vi "Generate Rotation Matrix.vi"(1 "Angle":dbl) -> (0 "Rotation Matrix":T1)   [LabVIEW 2019, in "Referential.lvclass"]
uses:
  Referential.lvclass
  <vilib>/Analysis/Matrix/Datatypes/RealMatrix.ctl
  <vilib>/Analysis/Matrix/NI_Matrix.lvlib
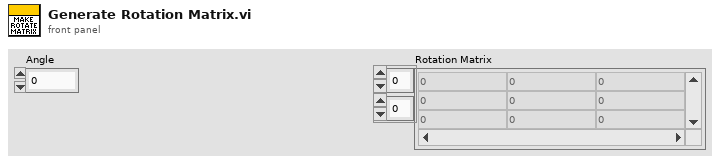
[diagram p1: front panel]
types:
  T1 = typedef "NI_Matrix.lvlib/RealMatrix.ctl" = dbl[][]
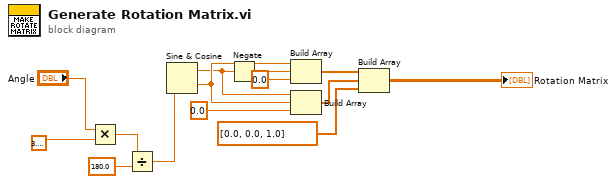
[diagram p0: block diagram]
diagram:
  n1 = Multiply(x="Angle", y=3.141592653589793) -> (x*y=w4:dbl)
  n2 = Divide(x=w4, y=180.0) -> (x/y=w1:dbl)
  n3 = Sine & Cosine(0:w1) -> (1:w10:dbl, 2:w11:dbl)
  n4 = Negate(x=w10) -> (-x=w14:dbl)
  n5 = Build Array(w11, w14, 0.0 ("element")) -> (w9:dbl[])
  n6 = Build Array(w10, w11, 0.0 ("element")) -> (w7:dbl[])
  n7 = Build Array(w9, w7, dbl[] [0.0, 0.0, 1.0] ("element")) -> (→"Rotation Matrix":T1)
